vi "getAVGFilterStatus.vi"(8 "error in (no error)":errorcluster, 10 "Measurement Function (0: Current)":T2, 11 "Electrometer in":refnum<class "Electrometer.lvclass">) -> (0 "error out":errorcluster, 1 "queryOK?":bool, 2 "AVG Filter type":T1, 3 "Electrometer out":refnum<class "Electrometer.lvclass">)   [LabVIEW 2016, in "Electrometer.lvclass"]
doc: "Query specific filter status for measuremente mode"
uses:
  Electrometer.lvclass
  Modes.ctl
  AVG Filter type.ctl
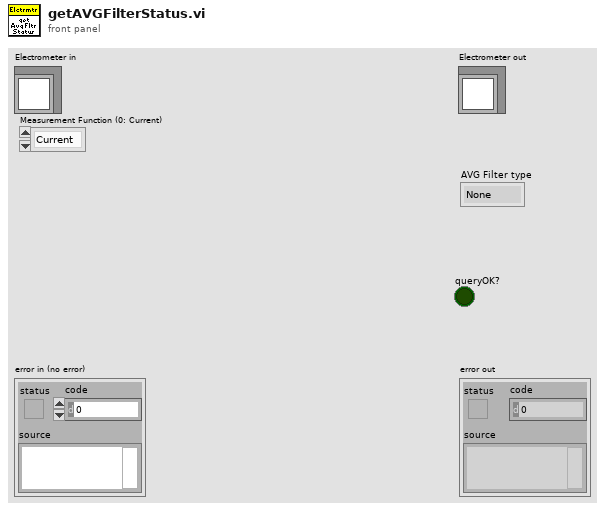
[diagram p1: front panel]
types:
  T1 = typedef "Electrometer.lvclass/AVG Filter type.ctl" = enum16{"None", "Scalar", "Advanced"}
  T2 = typedef "Electrometer.lvclass/Modes.ctl" = enum16{"Current", "Charge", "Voltage", "Resistance"}
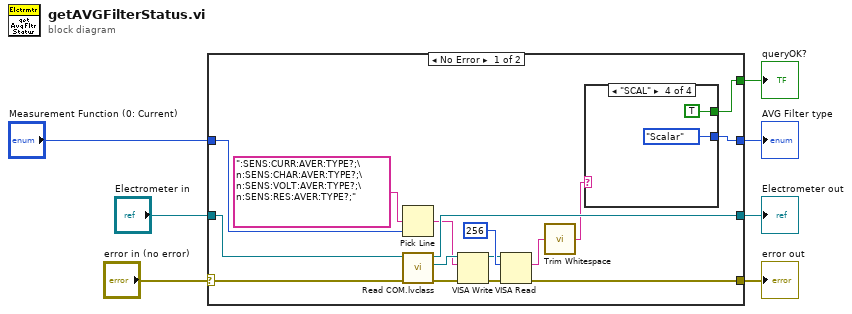
[diagram p0: block diagram]
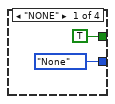
[diagram p2: hidden frame]
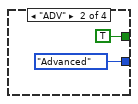
[diagram p3: hidden frame]
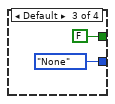
[diagram p4: hidden frame]
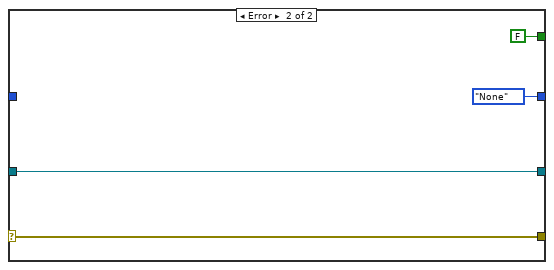
[diagram p5: hidden frame]
diagram:
  n1 = case shown="No Error" "error in (no error)" {
    selector: "error in (no error)" -> [w14 w35]
    tunnel: [w17 w35] -> w6
    tunnel: [w13 w34] -> w4
    tunnel: "Electrometer in" -> [w15 w34]
    tunnel: "Measurement Function (0: Current)" -> [w21 _]
    tunnel: [w16 FALSE] -> w3
    tunnel: [w10 AVG_Filter_type."None" ("AVG Filter type")] -> w1
    frame No Error {
      n2 = Pick Line(multi-line string=":SENS:CURR:AVER:TYPE?;\n:SENS:CHAR:AVER:TYPE?;\n:SENS:VOLT:AVER:TYPE?;\n:SENS:RES:AVER:TYPE?;", line index=w21) -> (output string=w11:string)  [unwired: 1 in]
      n3 = call "Read COM.lvclass.vi"("error in (no error)"=w14, "Electrometer in"=w15) -> ("error out"=w12:errorcluster, "VISA"=w23:refnum<visa-resource-name>, "Electrometer out"=w13:refnum<class "Electrometer.lvclass">)  [unwired: 7 in]
      n4 = VISA Write(VISA resource name=w23, write buffer=w11, error in (no error)=w12) -> (VISA resource name out=w19:refnum<visa-resource-name>, error out=w18:errorcluster)  [unwired: 1 out]
      n5 = VISA Read(VISA resource name=w19, byte count=u32 256, error in (no error)=w18) -> (read buffer=w9:string, error out=w17:errorcluster)  [unwired: 2 out]
      n6 = call <vilib>:"Trim Whitespace.vi"("string"=w9) -> ("trimmed string"=w8:string)  [unwired: 1 in]
      n7 = case shown="\"SCAL\"" w8 {
        tunnel: [AVG_Filter_type."None" ("AVG Filter type") AVG_Filter_type."Advanced" ("AVG Filter type") AVG_Filter_type."None" ("AVG Filter type") AVG_Filter_type."Scalar" ("AVG Filter type")] -> w10
        tunnel: [TRUE TRUE FALSE TRUE] -> w16
        frame "NONE" {
        }
        frame "ADV" {
        }
        frame Default {
        }
        frame "SCAL" {
        }
      }
    }
    frame Error {
    }
  }
  "error out" <- w6
  "Electrometer out" <- w4
  "queryOK?" <- w3
  "AVG Filter type" <- w1
